vi "Load parameters.vi"(8 "error in":errorcluster, 11 "INI data":T1) -> (0 "error out":errorcluster, 3 "INI data out":T1)   [LabVIEW 2014]
uses:
  Controls/INI config.ctl
  <vilib>/Utility/config.llb/Read Key (Double).vi
  <vilib>/Utility/config.llb/NI_LVConfig.lvlib
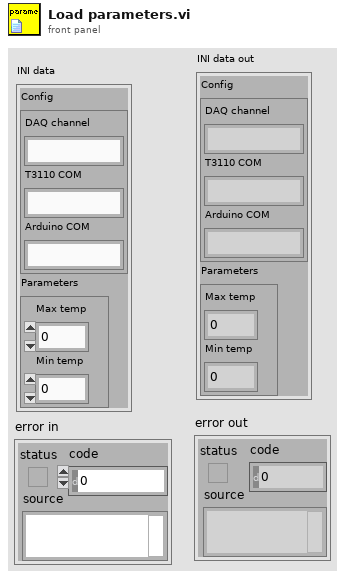
[diagram p1: front panel]
types:
  T1 = typedef "INI config.ctl" = cluster{"Config":cluster{"DAQ channel":string, "T3110 COM":string, "Arduino COM":string}, "Parameters":cluster{"Max temp":dbl, "Min temp":dbl}}
  T2 = typedef "NI_LVConfig.lvlib/Config Data RefNum.ctl" = refnum<k1>
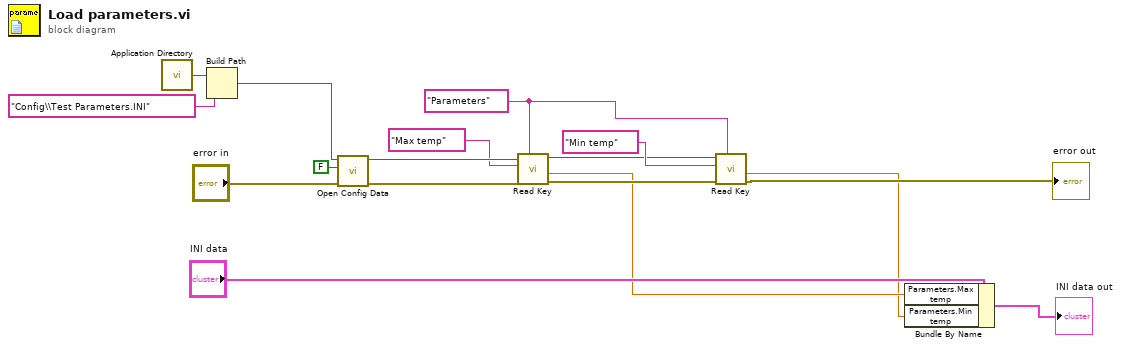
[diagram p0: block diagram]
diagram:
  w3 = "Parameters" ("section")
  n1 = call <vilib>:"Application Directory.vi"() -> ("Application Directory"=w12:path)
  n2 = Build Path(base path=w12, name or relative path="Config\\Test Parameters.INI") -> (appended path=w10:path)
  n3 = call <vilib>:"Open Config Data.vi"("error in (no error)"="error in", "create file if necessary (T)"=FALSE, "configuration file path"=w10) -> ("error out"=w14:errorcluster, "refnum"=w16:T2)  [unwired: 6 in, 1 out]
  n4 = call-poly <vilib>:"Read Key.vi"("section"=w3, "error in (no error)"=w14, "key"="Max temp", "refnum"=w16) -> ("error out"=w8:errorcluster, "value"=w2:dbl, "refnum out"=w5:T2)  [unwired: 4 in, 1 out]
  n5 = call-poly <vilib>:"Read Key.vi"("section"=w3, "error in (no error)"=w8, "key"="Min temp", "refnum"=w5) -> ("error out"=→"error out":errorcluster, "value"=w1:dbl)  [unwired: 4 in, 2 out]
  n6 = Bundle By Name(cluster="INI data", "Parameters.Max temp"=w2, "Parameters.Min temp"=w1) -> (→"INI data out":T1)
